vi "Is Instrument in Map.vi"(8 "error in":errorcluster, 10 "instrument type id":string, 11 "connection map in":refnum<class "Connection Map.lvclass">) -> (0 "error out":errorcluster, 2 "instrument in map":bool, 3 "connection map out":refnum<class "Connection Map.lvclass">)   [LabVIEW 2020, in "Measurement Plugin Session Management V1.lvlib" / "Connection Map.lvclass"]
uses:
  Connection Map.lvclass
  Connection Map.lvclass/Connection Map.ctl
  7369a05f-6fb4-4f66-8554-5e1198c88cf8.vi
  <vilib>/Comparison/Equal/Equal Functor/Equal Functor.lvclass
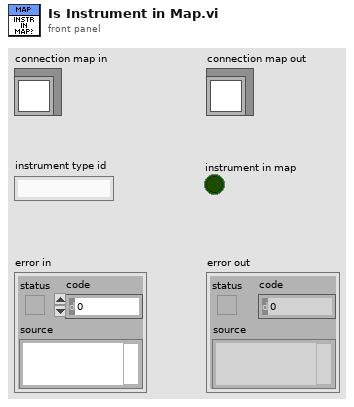
[diagram p1: front panel]
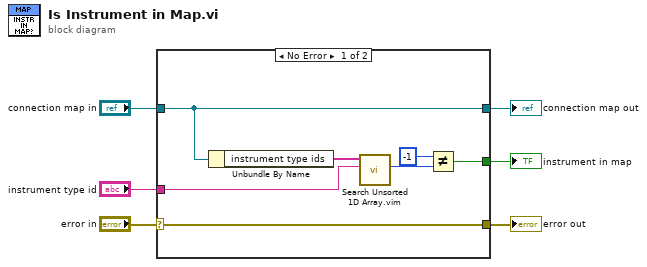
[diagram p0: block diagram]
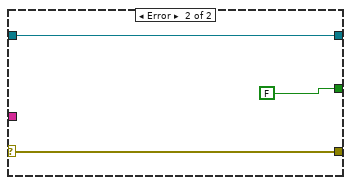
[diagram p2: hidden frame]
diagram:
  n1 = case shown="No Error" "error in" {
    selector: "error in" -> [w13 w16]
    tunnel: [w13 w16] -> w5
    tunnel: [w12 w15] -> w3
    tunnel: "connection map in" -> [w12 w15]
    tunnel: "instrument type id" -> [w10 _]
    tunnel: [w7 FALSE ("key not found?")] -> w1
    frame No Error {
      n2 = Unbundle By Name(w12) -> ("instrument type ids"=w11:string[])
      n3 = call "Search Unsorted 1D Array.vim"("element"=w10, "unsorted 1D array"=w11) -> ("index of element"=w9:i32)  [unwired: 9 in]
      n4 = Not Equal?(x=-1, y=w9) -> (x != y?=w7:bool)
    }
    frame Error {
    }
  }
  "error out" <- w5
  "connection map out" <- w3
  "instrument in map" <- w1
